vi "Write Settings to File.vi"(8 "error in (no error)":errorcluster, 10 "Settings Data":T1, 11 "appended path":path) -> (0 "error out":errorcluster)   [LabVIEW 2015, in "VI App Store.lvlib" / "VIStore.lvclass"]
uses:
  VIStore.lvclass
  Classes/Settings Item/Settings Data.ctl
  <vilib>/Utility/config.llb/Write Key (Path).vi
  <vilib>/Utility/config.llb/Write Key (Boolean).vi
  <vilib>/Utility/config.llb/NI_LVConfig.lvlib
  Classes/Settings Item/Settings.lvclass
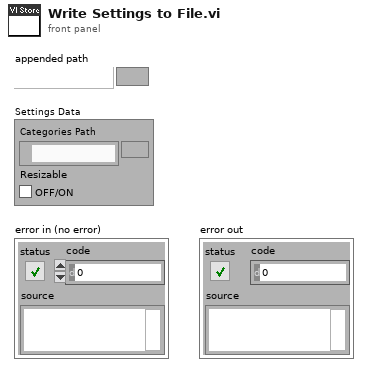
[diagram p1: front panel]
types:
  T1 = typedef "Item Actor.lvlib/Settings.lvclass/Settings Data.ctl" = cluster{"Categories Path":path, "Resizable":bool}
  T2 = typedef "NI_LVConfig.lvlib/Config Data RefNum.ctl" = refnum<k1>
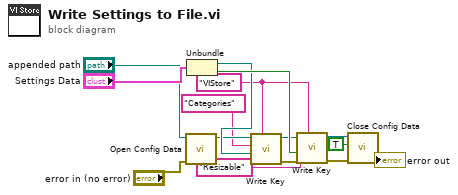
[diagram p0: block diagram]
diagram:
  w5 = "VIStore" ("section")
  n1 = call <vilib>:"Open Config Data.vi"("error in (no error)"="error in (no error)", "configuration file path"="appended path") -> ("error out"=w2:errorcluster, "refnum"=w9:T2)  [unwired: 7 in, 1 out]
  n2 = Unbundle("Settings Data") -> ("Categories Path"=w11:path, "Resizable"=w12:bool)
  n3 = call-poly <vilib>:"Write Key.vi"("section"=w5, "error in (no error)"=w2, "value"=w11, "key"="Categories", "refnum"=w9) -> ("error out"=w3:errorcluster, "refnum out"=w4:T2)  [unwired: 4 in, 1 out]
  n4 = call-poly <vilib>:"Write Key.vi"("section"=w5, "error in (no error)"=w3, "value"=w12, "key"="Resizable", "refnum"=w4) -> ("error out"=w13:errorcluster, "refnum out"=w10:T2)  [unwired: 4 in, 1 out]
  n5 = call <vilib>:"Close Config Data.vi"("error in (no error)"=w13, "write file if changed (T)"=TRUE, "refnum"=w10) -> ("error out"=→"error out":errorcluster)  [unwired: 7 in, 1 out]
